vi "ad digital out.vi"(7 "data":u32, 8 "error in (no error)":errorcluster, 10 "cha":i32, 11 "adh":i32) -> (0 "error out":errorcluster, 3 "function return":i32)   [LabVIEW 2021, in "libad4.lvlib"]
doc: "LIBAD4 function: ad_digital_out (int32_t adh, int32_t cha, uint32_t data);\n\nThis auxiliary function calls ad_discrete_out() with the channel number AD_CHA_TYPE_DIGITAL_IO|cha."
uses:
  <userlib>/libad4/libad4.lvlib
  <userlib>/libad4/libad4.dll
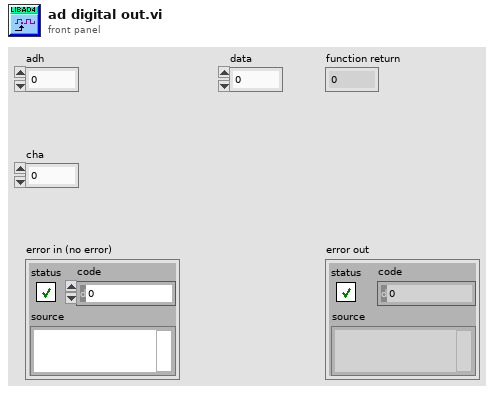
[diagram p1: front panel]
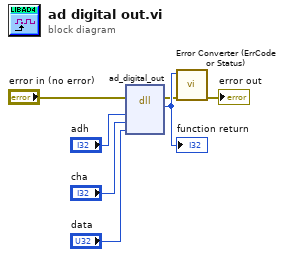
[diagram p0: block diagram]
diagram:
  n1 = dll-call lib="C:/Program Files/National Instruments/LabVIEW 2021/user.lib/libad4/libad4.*" fn="ad_digital_out"(error in="error in (no error)", "adh"="adh", "cha"="cha", "data"="data") -> (error out=w2:errorcluster, w7:i32)  [unwired: 5 in, 1 out]
  "function return" <- w7
  n2 = call <userlib>:"Error Converter (ErrCode or Status).vi"("error in (no error)"=w2, "error code"=w7) -> ("error out"=→"error out":errorcluster)  [unwired: 9 in]
